vi "getCurveFromString.vi"() -> ()   [LabVIEW 2017]
uses:
  f02d8b0b-6068-4eeb-8014-3bb825c9339c.vi
  <vilib>/Array/Sort 2D Array - Pop Stack.vi
  <vilib>/Array/Sort 2D Array - Push Stack.vi
  <vilib>/regexp/Match Regular Expression.xnode
panel:
  in  "字符串行":i32
  in  "输入字符串":string
  out "Rx":dbl[](array[numeric])
  in  "理论 K":dbl
  in  "R5-1":dbl
  out "曲线信息":string
  out "结果簇":cluster{dbl[], dbl[]}[](array[cluster])
  in  "传感器索引（1开始）":i32
  in  "检定次数":i32
  in  "正tmp":dbl[][](array[numeric])
  in  "反tmp":dbl[][](array[numeric])
  in  "压力点个数":i32
  in  "数据":string[][](array[string])
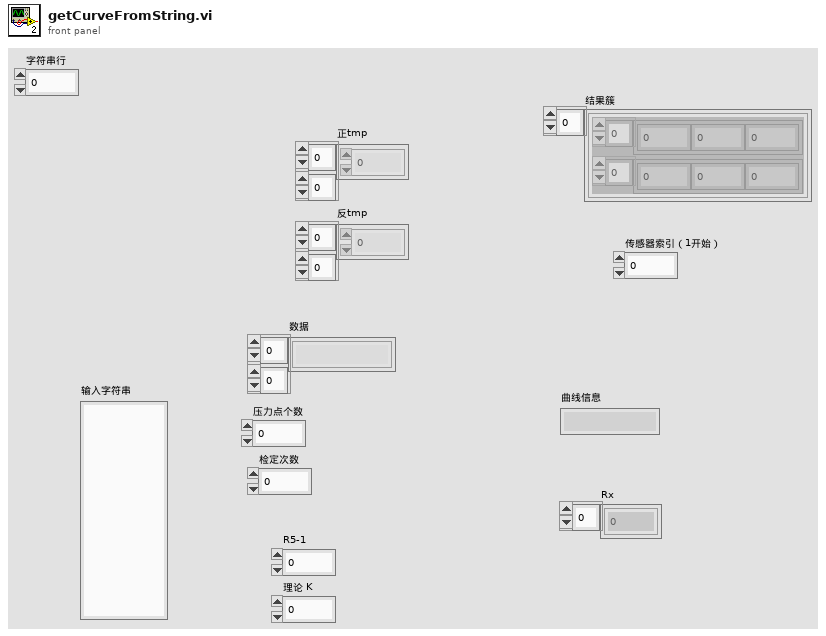
[diagram p1: front panel]
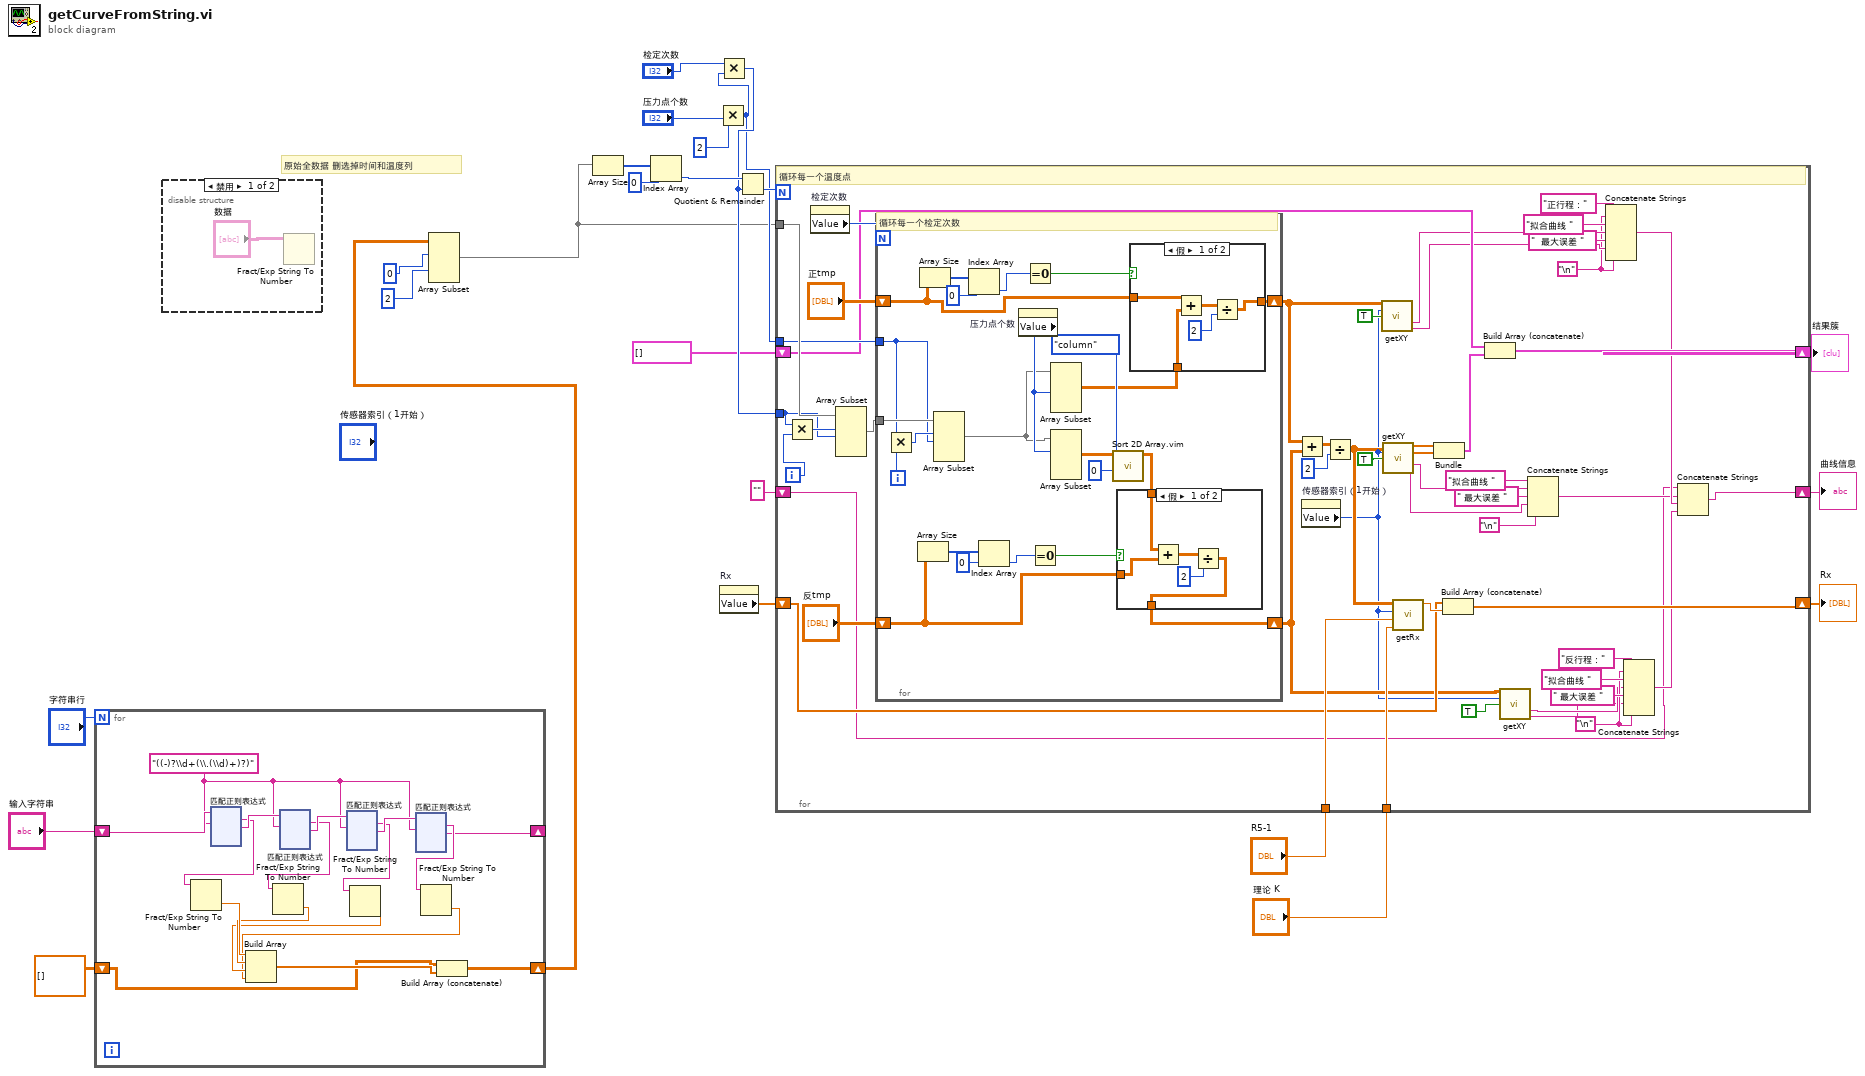
[diagram p0: block diagram]
diagram:
  # "原始全数据 删选掉时间和温度列"
  n1 = for {
    N: "字符串行" -> [_]
    shift-right: [w36] -> w1
    shift-left: dbl[][] [] -> [w35]
    shift-right: [w26] -> _
    shift-left: "输入字符串" -> [w34]
    w25 = "((-)?\\d+(\\.(\\d)+)?)"
    n2 = xnode "匹配正则表达式"("输入字符串"=w34, "正则表达式"=w25) -> ("所有匹配"=w30:string, "匹配之后"=w33:string)  [unwired: 4 in, 3 out]
    n3 = Fract/Exp String To Number(string=w30) -> (number=w41:dbl)  [unwired: 3 in, 1 out]
    n4 = xnode "匹配正则表达式"("输入字符串"=w33, "正则表达式"=w25) -> ("所有匹配"=w29:string, "匹配之后"=w32:string)  [unwired: 4 in, 3 out]
    n5 = Fract/Exp String To Number(string=w29) -> (number=w40:dbl)  [unwired: 3 in, 1 out]
    n6 = xnode "匹配正则表达式"("输入字符串"=w32, "正则表达式"=w25) -> ("所有匹配"=w28:string, "匹配之后"=w31:string)  [unwired: 4 in, 3 out]
    n7 = Fract/Exp String To Number(string=w28) -> (number=w39:dbl)  [unwired: 3 in, 1 out]
    n8 = xnode "匹配正则表达式"("输入字符串"=w31, "正则表达式"=w25) -> ("所有匹配"=w27:string, "匹配之后"=w26:string)  [unwired: 4 in, 3 out]
    n9 = Fract/Exp String To Number(string=w27) -> (number=w38:dbl)  [unwired: 3 in, 1 out]
    n10 = Build Array(w41, w40, w39, w38) -> (w37:dbl[])
    n11 = Build Array (concatenate)(w35, w37) -> (w36:dbl[][])
  }
  n12 = disable-structure shown="禁用" {
    frame Disabled {
      n13 = Fract/Exp String To Number(string="数据") -> ()  [unwired: 3 in, 2 out]
    }
    frame Enabled {
    }
  }
  n14 = Array Subset(array=w1, index (row)=0 ("长度"), index (col)=2 ("索引")) -> (w11:dbl[][])  [unwired: 2 in]
  n15 = Array Size(array=w11) -> (size(s)=w19:i32[])
  n16 = Index Array(array=w19, index=0 ("索引")) -> (element=w17:i32)
  n17 = Multiply(x=2, y="压力点个数") -> (x*y=w14:i32)
  n18 = Multiply(x="检定次数", y=w14) -> (x*y=w15:i32)
  n19 = property on="Rx" class="Arr (严格)"() -> ("Value"=w6:dbl[])  [unwired: 2 in, 2 out]
  n20 = Quotient & Remainder(x=w17, y=w15) -> (floor(x/y)=w20:i32)  [unwired: 1 out]
  n21 = for "循环每一个温度点" {
    N: w20 -> [_]
    tunnel: w11 -> [w548]
    tunnel: w15 -> [w545]
    tunnel: w14 -> [w542]
    shift-right: [w535] -> w12
    shift-left: cluster{dbl[], dbl[]}[] [] -> [w540]
    shift-right: [w500] -> w10
    shift-left: "" -> [w499]
    tunnel: "R5-1" -> [w525]
    tunnel: "理论 K" -> [w524]
    shift-right: [w521] -> w7
    shift-left: w6 -> [w522]
    i -> [w547]
    w506 = "\n"
    w513 = "\n"
    # "循环每一个温度点"
    n22 = Multiply(x=w545, y=w547) -> (x*y=w546:i32)
    n23 = property on="检定次数" class="DigNum (严格)"() -> ("Value"=w544:i32)  [unwired: 2 in, 2 out]
    n24 = Array Subset(array=w548, index (row)=w546, length (row)=w545) -> (w543:dbl[][])  [unwired: 2 in]
    n25 = for {
      N: w544 -> [_]
      tunnel: w543 -> [w567]
      tunnel: w542 -> [w564]
      shift-right: [w558] -> w520
      shift-left: "正tmp" -> [w557]
      shift-right: [w550] -> w512
      shift-left: "反tmp" -> [w549]
      i -> [w566]
      # "循环每一个检定次数"
      n26 = Multiply(x=w564, y=w566) -> (x*y=w565:i32)
      n27 = Array Size(array=w549) -> (size(s)=w556:i32[])
      n28 = Array Size(array=w557) -> (size(s)=w562:i32[])
      n29 = Array Subset(array=w567, index (row)=w565, length (row)=w564) -> (w563:dbl[][])  [unwired: 2 in]
      n30 = Index Array(array=w562, index=0 ("索引")) -> (element=w560:i32)
      n31 = Index Array(array=w556, index=0 ("索引")) -> (element=w554:i32)
      n32 = property on="压力点个数" class="DigNum (严格)"() -> ("Value"=w571:i32)  [unwired: 2 in, 2 out]
      n33 = Equal To 0?(x=w560) -> (x = 0?=w559:bool)
      n34 = Equal To 0?(x=w554) -> (x = 0?=w553:bool)
      n35 = Array Subset(array=w563, length (row)=w571) -> (w552:dbl[][])  [unwired: 3 in]
      n36 = Array Subset(array=w563, index (row)=w571) -> (w568:dbl[][])  [unwired: 3 in]
      n37 = call "Sort 2D Array.vim"("index"=0, "dimension to index (column)"=enum16{"column", "row"}."column", "2D array"=w568) -> ("sorted 2D array"=w551:dbl[][])  [unwired: 7 in, 1 out]
      n38 = case shown="假" w553 {
        tunnel: w551 -> [w575 w577]
        tunnel: [w572 w577] -> w550
        tunnel: w549 -> [w576 _]
        frame False {
          n39 = Add(x=w575, y=w576) -> (x+y=w574:dbl[][])
          n40 = Divide(x=w574, y=2) -> (x/y=w572:dbl[][])
        }
        frame True {
        }
      }
      n41 = case shown="假" w559 {
        tunnel: w552 -> [w580 w583]
        tunnel: [w578 w583] -> w558
        tunnel: w557 -> [w579 _]
        frame False {
          n42 = Add(x=w579, y=w580) -> (x+y=w582:dbl[][])
          n43 = Divide(x=w582, y=2) -> (x/y=w578:dbl[][])
        }
        frame True {
        }
      }
    }
    n44 = Add(x=w520, y=w512) -> (x+y=w538:dbl[][])
    n45 = property on="传感器索引（1开始）" class="DigNum (严格)"() -> ("Value"=w511:i32)  [unwired: 2 in, 2 out]
    n46 = Divide(x=w538, y=2) -> (x/y=w526:dbl[][])
    n47 = call "getXY.vi"("数据"=w520, "传感器索引"=w511, "是否需要计算拟合曲线"=TRUE) -> ("拟合曲线"=w516:string, "最大误差率"=w515:string)  [unwired: 5 in, 6 out]
    n48 = call "getXY.vi"("数据"=w526, "传感器索引"=w511, "是否需要计算拟合曲线"=TRUE) -> ("x"=w533:dbl[], "y"=w532:dbl[], "拟合曲线"=w531:string, "最大误差率"=w528:string)  [unwired: 5 in, 4 out]
    n49 = call "getRx.vi"("理论 K"=w524, "R5-1"=w525, "传感器索引"=w511, "数据"=w526) -> ("Rx"=w523:dbl)  [unwired: 7 in]
    n50 = Bundle("x"=w533, "y"=w532) -> (w536:cluster{"x":dbl[], "y":dbl[]})  [unwired: 1 in]
    n51 = Build Array (concatenate)(w522, w523) -> (w521:dbl[])
    n52 = Build Array (concatenate)(w540, w536) -> (w535:cluster{"x":dbl[], "y":dbl[]}[])
    n53 = call "getXY.vi"("数据"=w512, "传感器索引"=w511, "是否需要计算拟合曲线"=TRUE) -> ("拟合曲线"=w505:string, "最大误差率"=w504:string)  [unwired: 5 in, 6 out]
    n54 = Concatenate Strings("拟合曲线 " ("字符串"), w531, " 最大误差 " ("字符串"), w528, "\n") -> (w501:string)
    n55 = Concatenate Strings("正行程：" ("字符串"), w513, "拟合曲线 " ("字符串"), w516, "  最大误差 " ("字符串"), w515, w513) -> (w502:string)
    n56 = Concatenate Strings("反行程：" ("字符串"), w506, "拟合曲线 " ("字符串"), w505, " 最大误差 " ("字符串"), w504, w506) -> (w503:string)
    n57 = Concatenate Strings(w499, w501, w502, w503) -> (w500:string)
  }
  "结果簇" <- w12
  "曲线信息" <- w10
  "Rx" <- w7
